vi "Untitled 2 (SubVI).vi"(10 "x":i16, 11 "x 2":dbl) -> (2 "s? t:f 3":dbl, 3 "s? t:f":dbl)   [LabVIEW 2015]
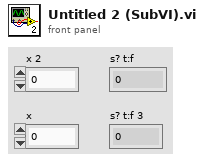
[diagram p1: front panel]
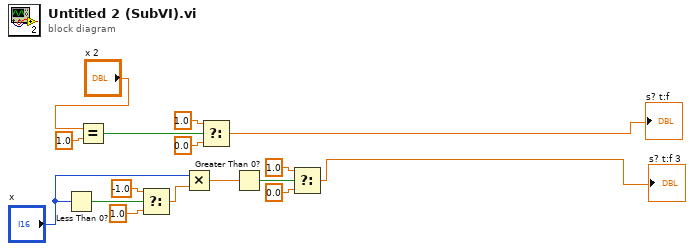
[diagram p0: block diagram]
diagram:
  n1 = Less Than 0?(x="x") -> (x < 0?=w1:bool)
  n2 = Equal?(x="x 2", y=1.0) -> (x = y?=w11:bool)
  n3 = Select(t=-1.0, s=w1, f=1.0) -> (s? t:f=w4:dbl)
  n4 = Multiply(x="x", y=w4) -> (x*y=w5:dbl)
  n5 = Select(t=1.0, s=w11, f=0.0) -> (s? t:f=→"s? t:f":dbl)
  n6 = Greater Than 0?(x=w5) -> (x > 0?=w6:bool)
  n7 = Select(t=1.0, s=w6, f=0.0) -> (s? t:f=→"s? t:f 3":dbl)
